vi "读取各参数配置.vi"(8 "error in (no error)":errorcluster, 10 "参数":string(combo)="参考灵敏度", 11 "NI_report输入":refnum<class "NI_report.lvclass">) -> (0 "error out":errorcluster, 2 "设置":string[][](array[string]), 3 "report out":refnum<class "NI_report.lvclass">, 5 "测量点数":i32)   [LabVIEW 2015]
uses:
  <vilib>/Utility/NIReport.llb/NI_report.lvclass
  <vilib>/addons/_office/excel.llb/Excel Get Data ([str]).vi
  <vilib>/addons/_office/NI_ReportGenerationToolkit.lvlib
  <vilib>/Utility/NIReport.llb/Excel/NI_Excel.lvclass
panel:
  in  "模板":path=path "C:/Documents and Settings/Administrator/Desktop/加速度传感器自动化程序——田晓涛/原始记录模板/单向电荷型加速度传感器10-5000.xls"
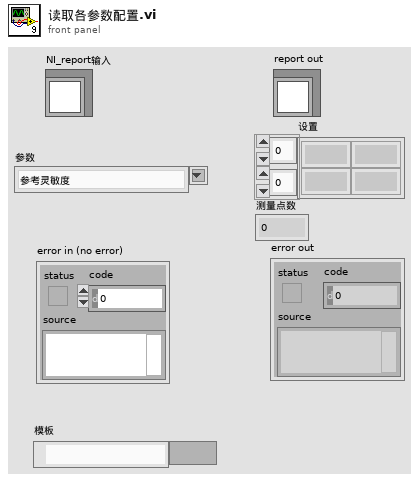
[diagram p1: front panel]
types:
  T1 = enum16{"Standard Report", "HTML", "Word", "Excel"}
  T2 = enum16{"maximized", "minimized", "normal", "no change"}
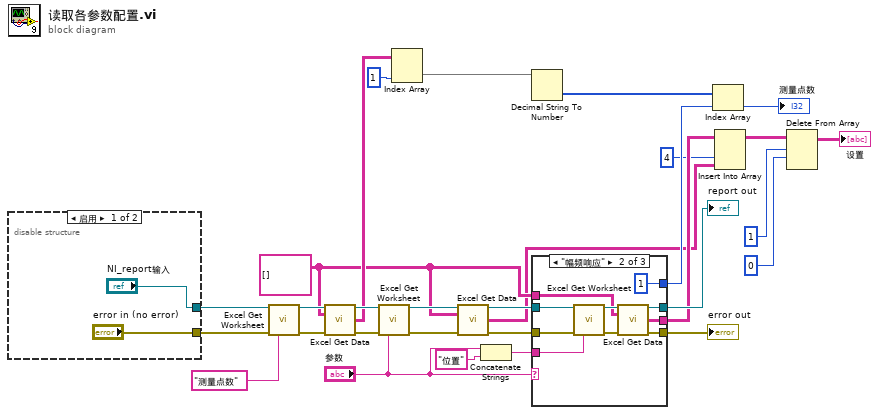
[diagram p0: block diagram]
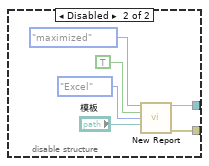
[diagram p2: hidden frame]
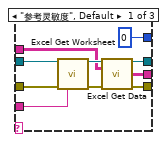
[diagram p3: hidden frame]
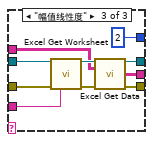
[diagram p4: hidden frame]
diagram:
  w8 = string[][] [] ("data type")
  n1 = disable-structure shown="启用" {
    disable-tunnel: ["NI_report输入" w34] -> w26
    disable-tunnel: ["error in (no error)" w33] -> w25
    frame Enabled {
    }
    frame Disabled {
      n2 = call <vilib>:"New Report.vi"("window state (normal)"=T2."maximized", "display alerts? (F)"=TRUE, "report type"=T1."Excel", "template (empty)"="模板") -> ("report out"=w34:refnum<class "NI_report.lvclass">, "error out"=w33:errorcluster)  [unwired: 10 in]
    }
  }
  n3 = call <vilib>:"Excel Get Worksheet.vi"("report in"=w26, "error in (no error)"=w25, "name (\"\")"="测量点数" ("name (\"\")")) -> ("report out"=w24:refnum<class "NI_report.lvclass">, "error out"=w21:errorcluster)  [unwired: 11 in]
  n4 = call-poly <vilib>:"Excel Get Data.vi"("report in"=w24, "data type"=w8, "error in (no error)"=w21) -> ("report out"=w23:refnum<class "NI_report.lvclass">, "data"=w19:string[][], "error out"=w22:errorcluster)  [unwired: 10 in]
  n5 = call <vilib>:"Excel Get Worksheet.vi"("report in"=w23, "error in (no error)"=w22, "name (\"\")"="参数") -> ("report out"=w29:refnum<class "NI_report.lvclass">, "error out"=w30:errorcluster)  [unwired: 11 in]
  n6 = Index Array(array=w19, index (col)=1 ("禁用的索引 (列)")) -> (element=w17:string[])  [unwired: 1 in]
  n7 = call-poly <vilib>:"Excel Get Data.vi"("report in"=w29, "data type"=w8, "error in (no error)"=w30) -> ("report out"=w11:refnum<class "NI_report.lvclass">, "data"=w4:string[][], "error out"=w10:errorcluster)  [unwired: 10 in]
  n8 = Concatenate Strings("参数", "位置" ("字符串")) -> (w9:string)
  n9 = Decimal String To Number(string=w17) -> (number=w16:i32[])  [unwired: 2 in, 1 out]
  n10 = case shown="\"幅频响应\"" "参数" {
    tunnel: [0 1 2] -> w15
    tunnel: w11 -> [w45 w57 w67]
    tunnel: w10 -> [w44 w56 w66]
    tunnel: w9 -> [w40 w55 w65]
    tunnel: [w43 w52 w62] -> w7
    tunnel: [w42 w51 w61] -> w6
    tunnel: w8 -> [w39 w50 w60]
    tunnel: [w46 w49 w59] -> w5
    frame "参考灵敏度", Default {
      n11 = call <vilib>:"Excel Get Worksheet.vi"("report in"=w45, "error in (no error)"=w44, "name (\"\")"=w40) -> ("report out"=w41:refnum<class "NI_report.lvclass">, "error out"=w47:errorcluster)  [unwired: 11 in]
      n12 = call-poly <vilib>:"Excel Get Data.vi"("report in"=w41, "data type"=w39, "error in (no error)"=w47) -> ("report out"=w43:refnum<class "NI_report.lvclass">, "data"=w46:string[][], "error out"=w42:errorcluster)  [unwired: 10 in]
    }
    frame "幅频响应" {
      n13 = call <vilib>:"Excel Get Worksheet.vi"("report in"=w57, "error in (no error)"=w56, "name (\"\")"=w55) -> ("report out"=w53:refnum<class "NI_report.lvclass">, "error out"=w54:errorcluster)  [unwired: 11 in]
      n14 = call-poly <vilib>:"Excel Get Data.vi"("report in"=w53, "data type"=w50, "error in (no error)"=w54) -> ("report out"=w52:refnum<class "NI_report.lvclass">, "data"=w49:string[][], "error out"=w51:errorcluster)  [unwired: 10 in]
    }
    frame "幅值线性度" {
      n15 = call <vilib>:"Excel Get Worksheet.vi"("report in"=w67, "error in (no error)"=w66, "name (\"\")"=w65) -> ("report out"=w64:refnum<class "NI_report.lvclass">, "error out"=w63:errorcluster)  [unwired: 11 in]
      n16 = call-poly <vilib>:"Excel Get Data.vi"("report in"=w64, "data type"=w60, "error in (no error)"=w63) -> ("report out"=w62:refnum<class "NI_report.lvclass">, "data"=w59:string[][], "error out"=w61:errorcluster)  [unwired: 10 in]
    }
  }
  "report out" <- w7
  "error out" <- w6
  n17 = Index Array(array=w16, index=w15) -> (element=→"测量点数":i32)
  n18 = Insert Into Array(array=w5, index (col)=4 ("禁用的索引 (列)"), new element=w4) -> (w2:string[][])  [unwired: 1 in]
  n19 = Delete From Array(array=w2, length=1 ("长度"), index (row)=0 ("索引 (行)")) -> (array with subset deleted=→"设置":string[][])  [unwired: 1 in, 1 out]
